vi "Read Input DBL Values.vi"(8 "error in (no error)":errorcluster, 9 "number of registers":u16, 10 "starting address":u16, 11 "standard data model in":refnum<class "ELAN Data Model.lvclass">) -> (0 "error out":errorcluster, 2 "Values":dbl[](array[numeric]), 3 "standard sata model out":refnum<class "ELAN Data Model.lvclass">)   [LabVIEW 2021, in "ELAN Data Model.lvclass"]
doc: "Reads N holding registers from the device model, starting at register M."
uses:
  ELAN Data Model.lvclass
  ELAN Data Model.lvclass/ELAN Data Model.ctl
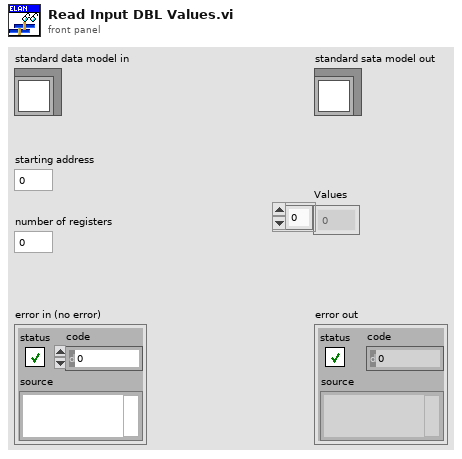
[diagram p1: front panel]
types:
  T1 = typedef "ELAN Data Model.lvclass/Data Model.ctl" = cluster{"UTC":u64, "Value":T2[]}
  T2 = typedef "ELAN Data Model.lvclass/Value full.ctl" = cluster{"Value":cluster{"Value":sgl, "units":T3, "component":T4}, "channel state":T5, "collective state":errorcluster}
  T3 = typedef "ELAN PDU.lvclass/Elan units.ctl" = enum16{"Invalid", "no dimension", "ppm", "ppb", "vpm", "ppm C1", "ppm C3", "ppm C6", "mg C/m3", "mg/m3", "%", "% vol", "% of measuring range", "% saturation", "%/°C", "%/K", "% weight", "mV/pH", "mV/mbar", "nA/mbar", "S/m", "S/cm", "mS/m", "mS/cm", "ìS/m", "ìS/cm", "S", "min", "H", "Pa", "MA", "uV", "MV", "V", "mbar", "hPa", "Ml/min", "kOhm", "MOhm", "S1", "°C", "Hz", "pH", "ug/l", "mg/l", "l/min", "uA", "mg/dm3", "kPa", "kOhm*cm", "MOhm*cm", "°", "1/min", "1/m", "g/m3", "g/l", "% Vol C"}
  T4 = typedef "ELAN PDU.lvclass/Elan measured variable.ctl" = enum16{"Invalid", "no component", "CO", "CO2", "CH4 (Methan)", "C6H14 (Hexan)", "SO2", "NO", "NO2", "CHClF2 (R22)", "C3H8 (Propan)", "C4H10 (Butan)", "O2", "C5H12 (Pentan)", "CnHm (THC)", "P (process pressure)", "pH", "T (temperature)", "C2H4 (Ethen)", "C2H2 (Ethin)", "C3H6 (Propen)", "C4H6", "C4H8", "C2H6", "NH3 (Ammoniak)", "N2O", "C6H6 (Benzol)", "SF6", "CH3OH (Methanol)", "C2H5OH (Ethanol)", "CH2Cl2", "C2H4Cl2", "CH3Cl", "C2H4O", "H2O (water vapor)", "G/l (conductivity)", "C", "S", "N", "CF4", "COCl2 (phosgene)", "CHF3 (R23)", "C2F6 (R116)", "------ (self defined component)", "C2H3Cl", "H2 (Hydrogen)", "Ar", "He", "Cl2", "N2"}
  T5 = typedef "ELAN PDU.lvclass/Elan channel state.ctl" = enum16{"Invalid", "Warm-up", "Pause", "Standby", "Measure", "Zero calibration", "Adjust component slope", "Not yet defined1", "Adjust curve dip", "Adjust linearization sensitivity", "Adjust temperature compensation", "Adjust pressure compensation", "Adjust linearization zero", "Not yet defined2", "Autocal", "Adjust phase", "Zero calibration of O2 sensor", "Synchronous zero calibration", "Purging for synchronous zero calibration", "Adjust analog output", "Adjust analog input", "Autocal check"}
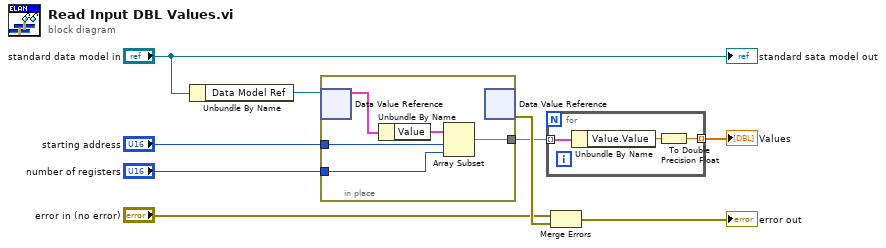
[diagram p0: block diagram]
diagram:
  n1 = Unbundle By Name("standard data model in") -> ("Data Model Ref"=w5:refnum<data-value>)
  n2 = in-place {
    in-place-border: [w14] -> w2
    in-place-border: "starting address" -> [w13]
    in-place-border: "number of registers" -> [w12]
    n3 = in-place-dvr #1(w5) -> (w11:T1)  [unwired: 1 out]
    n4 = Unbundle By Name(w11) -> ("Value"=w10:T2[])
    n5 = Array Subset(array=w10, index=w13, length=w12) -> (w14:T2[])
    n6 = in-place-dvr #1() -> (w4:errorcluster)  [unwired: 1 in, 1 out]
  }
  n7 = for {
    tunnel: w2 -> [w17] mode=indexing
    tunnel: [w15] -> w1 mode=indexing
    n8 = Unbundle By Name(w17) -> ("Value.Value"=w16:sgl)
    n9 = To Double Precision Float(number=w16) -> (double precision float=w15:dbl)
  }
  "Values" <- w1
  n10 = Merge Errors("error in (no error)", w4) -> (→"error out":errorcluster)
  "standard sata model out" <- "standard data model in"
